vi "Update Hall Calibration.vi"(8 "C":dbl, 9 "B":dbl, 10 "A":dbl) -> ()   [LabVIEW 2009, in "Varian Magnet.lvclass"]
doc: "Simple Pop-up GUI to make sure Hall Calibration Constants are set properly."
uses:
  Varian Magnet.lvclass
  Varian Constants.vi
panel:
  in  "Set & Continue":bool
  in  "Yes/No Button":bool
  out "C Old":dbl
  out "B Old":dbl
  out "A Old":dbl
  # "Do you want to replace\nthese calibration values\nwith these calibration \nvalues?"
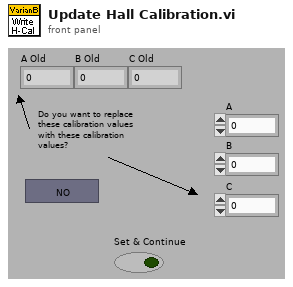
[diagram p1: front panel]
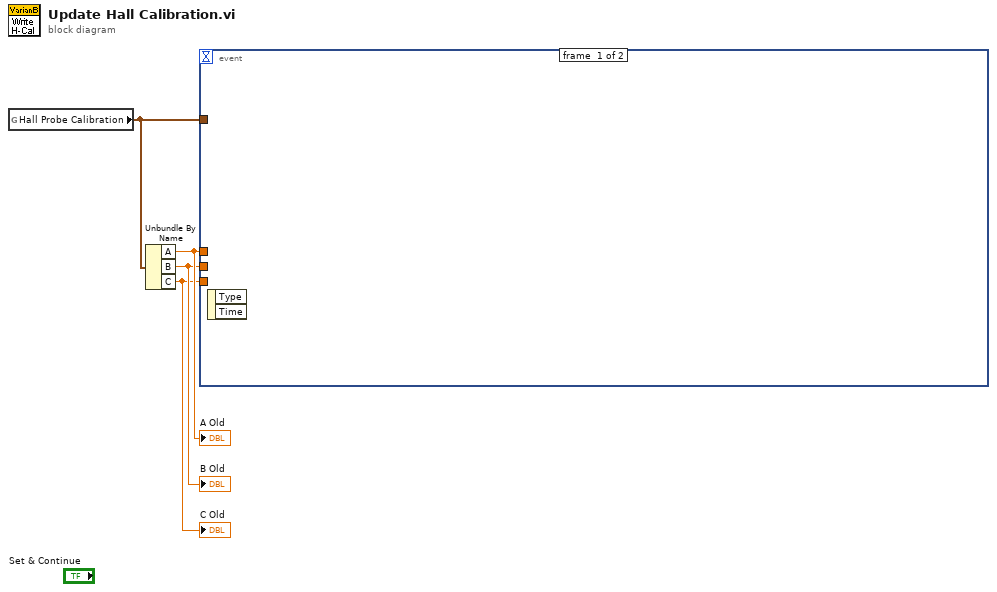
[diagram p0: block diagram]
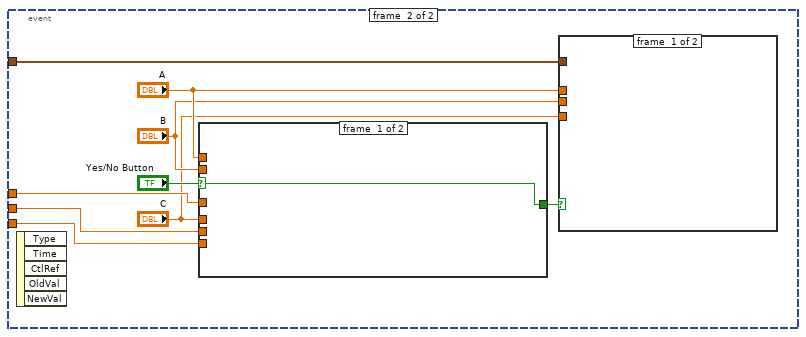
[diagram p2: hidden frame]
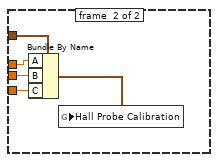
[diagram p3: hidden frame]
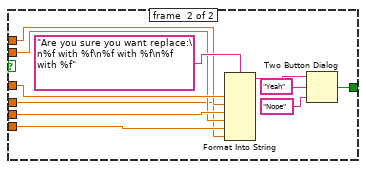
[diagram p4: hidden frame]
diagram:
  n1 = global read "Varian Constants.vi" "Hall Probe Calibration"() -> (w4:cluster{"A":dbl, "B":dbl, "C":dbl})
  n2 = Unbundle By Name(w4) -> ("A"=w3:dbl, "B"=w2:dbl, "C"=w1:dbl)
  "A Old" <- w3
  "B Old" <- w2
  "C Old" <- w1
  n3 = event shown="[1] \"Set & Continue\": Value Change" {
    selector: _ -> [_ _]
    dyn-events: _ -> [_ _]
    timeout: _ -> [_ _]
    tunnel: w4 -> [_ w11]
    tunnel: w3 -> [_ w10]
    tunnel: w2 -> [_ w9]
    tunnel: w1 -> [_ w8]
    event #0 {
      n4 = event-data() -> ()  [unwired: 1 in, 2 out]
    }
    event #1 {
      n5 = event-data() -> ()  [unwired: 1 in, 5 out]
      n6 = case shown="True" "Yes/No Button" {
        selector: "Yes/No Button" -> [w19 _]
        tunnel: [w19 w28] -> w12
        tunnel: w10 -> [_ w26]
        tunnel: w9 -> [_ w25]
        tunnel: w8 -> [_ w24]
        tunnel: "A" -> [_ w23]
        tunnel: "B" -> [_ w22]
        tunnel: "C" -> [_ w21]
        frame #0 {
        }
        frame #1 {
          n7 = Format Into String(format string="Are you sure you want replace:\n%f with %f\n%f with %f\n%f with %f" ("message"), w26, w23, w25, w22, w24, w21) -> (resulting string=w20:string)  [unwired: 2 in, 1 out]
          n8 = Two Button Dialog(message=w20, 1:"Nope" ("F button name (\"Cancel\")"), 2:"Yeah" ("T button name (\"OK\")")) -> (T button?=w28:bool)
        }
      }
      n9 = case shown="True" w12 {
        tunnel: w11 -> [_ w18]
        tunnel: "A" -> [_ w17]
        tunnel: "B" -> [_ w16]
        tunnel: "C" -> [_ w15]
        frame #0 {
        }
        frame #1 {
          n10 = Bundle By Name(cluster=w18, "A"=w17, "B"=w16, "C"=w15) -> (w14:cluster{"A":dbl, "B":dbl, "C":dbl})
          n11 = global write "Varian Constants.vi" "Hall Probe Calibration"(w14) -> ()
        }
      }
    }
  }
